vi "GetLineVoltages.vi"(9 "delta connection? (F)":bool, 11 "original voltages":fxp<+/-,24,10>[](array[numeric])=[0.0, 0.0, 0.0]) -> (3 "line or phase voltages":fxp<+/-,25,11>[](array[numeric]))   [LabVIEW 2017, in "MCSA_9065_API.lvlib"]
uses:
  <vilib>/addons/InsightCM/Devices/Shared/Mcsa/Fpga/McsaAcquire/subVIs/McsaAPI_9065/MCSA_9065_API.lvlib
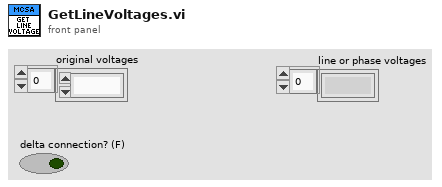
[diagram p1: front panel]
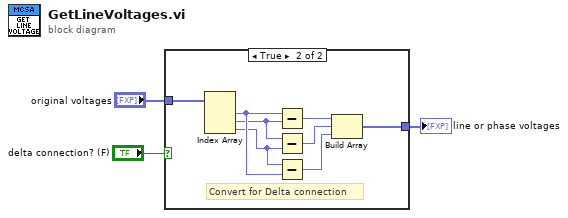
[diagram p0: block diagram]
diagram:
  n1 = case shown="True" "delta connection? (F)" {
    tunnel: [w4 w6] -> w3
    tunnel: "original voltages" -> [w4 w5]
    frame False {
      # "No action for Wye connection"
    }
    frame True {
      # "Convert for Delta connection"
      n2 = Index Array(array=w5) -> (element #1=w9:fxp<+/-,24,10>, element #2=w7:fxp<+/-,24,10>, element #3=w8:fxp<+/-,24,10>)  [unwired: 3 in]
      n3 = Subtract(x=w9, y=w7) -> (x-y=w10:fxp<+/-,25,11>)
      n4 = Subtract(x=w7, y=w8) -> (x-y=w11:fxp<+/-,25,11>)
      n5 = Subtract(x=w8, y=w9) -> (x-y=w12:fxp<+/-,25,11>)
      n6 = Build Array(w10, w11, w12) -> (w6:fxp<+/-,25,11>[])
    }
  }
  "line or phase voltages" <- w3
